vi "UHR-Fleezers Control (host) - 10.4.vi"() -> ()   [LabVIEW 2011] (continued)
        n819 = Select(t=w1240, s="+ phase (GI)", f="Phase adj. (GI)") -> (s? t:f=w1239:i16)
        n820 = Or(x="+ phase (GI)", y="- phase (GI)") -> (x .or. y?=w1235:bool)
        n821 = xnode "Read/Write Control"("FPGA VI Reference In"=w1242, "error in"=w1241, "Phase count adjustment (GI)"=w1239) -> ("FPGA VI Reference Out"=w1237:T19, "error out"=w1238:errorcluster)
        n822 = xnode "Read/Write Control"("FPGA VI Reference In"=w1237, "error in"=w1238, "+ phase (GI)"=w1235) -> ("error out"=w1236:errorcluster)  [unwired: 1 out]
      }
      event "Phase adj. (GI) 2", "+ phase (GI) 2", "- phase (GI) 2": Value Change {
        n823 = event-data() -> ()  [unwired: 7 out]
        n824 = Negate(x="Phase adj. (GI) 2") -> (-x=w1251:i16)
        n825 = Select(t=w1251, s="+ phase (GI) 2", f="Phase adj. (GI) 2") -> (s? t:f=w1250:i16)
        n826 = Or(x="+ phase (GI) 2", y="- phase (GI) 2") -> (x .or. y?=w1246:bool)
        n827 = xnode "Read/Write Control"("FPGA VI Reference In"=w1253, "error in"=w1252, "Phase count adjustment (GI) 2"=w1250) -> ("FPGA VI Reference Out"=w1248:T19, "error out"=w1249:errorcluster)
        n828 = xnode "Read/Write Control"("FPGA VI Reference In"=w1248, "error in"=w1249, "+ phase (GI) 2"=w1246) -> ("error out"=w1247:errorcluster)  [unwired: 1 out]
      }
      event "Phase adj. (Green FB)", "- phase (Green FB)", "+ phase (Green FB)": Value Change {
        n829 = event-data() -> ()  [unwired: 7 out]
        n830 = Negate(x="Phase adj. (Green FB)") -> (-x=w1262:i16)
        n831 = Select(t=w1262, s="+ phase (Green FB)", f="Phase adj. (Green FB)") -> (s? t:f=w1261:i16)
        n832 = Or(x="+ phase (Green FB)", y="- phase (Green FB)") -> (x .or. y?=w1257:bool)
        n833 = xnode "Read/Write Control"("FPGA VI Reference In"=w1264, "error in"=w1263, "Phase count adjustment (Green FB)"=w1261) -> ("FPGA VI Reference Out"=w1259:T19, "error out"=w1260:errorcluster)
        n834 = xnode "Read/Write Control"("FPGA VI Reference In"=w1259, "error in"=w1260, "+ phase (Green FB)"=w1257) -> ("error out"=w1258:errorcluster)  [unwired: 1 out]
      }
      event "Invert APD Gate", "APD Gate ON Count", "APD Gate OFF Count", "APD Gate", "APD Integration Time (s)", "APD 1 AO Mult.", "APD 2 AO Mult.", "On one out of X cycles": Value Change {
        n835 = event-data() -> ()  [unwired: 7 out]
        n836 = Add(x="GI Frequency, ON count", y="GI Frequency, OFF count") -> (x+y=w1268:u32)
        n837 = Add(x="APD Gate ON Count", y="APD Gate OFF Count") -> (x+y=w1281:u32)
        n838 = Multiply(x="On one out of X cycles", y=w1268) -> (x*y=w1265:u32)
        "Green FB Count" <- w1265
        n839 = Subtract(x=w1265, y="GI Frequency, ON count") -> (x-y=w1266:u32)
        n840 = Multiply(x=w1281, y="On one out of X cycles") -> (x*y=w1280:u32)
        n841 = Subtract(x=w1280, y="APD Gate ON Count") -> (x-y=w1279:u32)
        n842 = local read "DMA Update Period (s)"() -> (w1282:dbl)
        n843 = Multiply(x="APD Integration Time (s)", y=40000000.0) -> (x*y=w1287:dbl)
        n844 = Reciprocal(x="APD Integration Time (s)") -> (1/x=→"APD Acq Rate (Hz)":dbl)
        n845 = To Unsigned Long Integer(number=w1287) -> (unsigned 32bit integer=w1271:u32)
        "APD Int. Count" <- w1271
        n846 = xnode "Read/Write Control"("FPGA VI Reference In"=w1291, "error in"=w1290, "Invert APD Gate"="Invert APD Gate", "APD Gate ON Count"="APD Gate ON Count", "APD Gate OFF Count"=w1279, "APD Acq Rate Count"=w1271, "APD Gate Operating Mode"="APD Gate", "APD 1 AO scale factor"="APD 1 AO Mult.", "APD 2 AO scale factor"="APD 2 AO Mult.", "Green interlace ON count"="GI Frequency, ON count", "Green interlace OFF count"=w1266, "Green interlace ON count 2"="GI Frequency, ON count", "Green interlace OFF count 2"=w1266, "Green FB Count"=w1265) -> ("error out"=w1289:errorcluster)  [unwired: 1 out]
        n847 = Divide(x=w1282, y="APD Integration Time (s)") -> (x/y=w1285:dbl)
        n848 = Multiply(x=2.0, y=w1285) -> (x*y=w1284:dbl)
        n849 = local write "APD Samples/FIFO Acq."(w1285) -> ()
        n850 = local write "APD Elements/DMA read"(w1284) -> ()
      }
      event "Number of F/B Scans (AOD)", "Scan Speed (nm/s)", "Scan BD", "Initial delta (MHz)", "Step Size (nm)", "Scan Range (nm)": Value Change {
        w1353 = 123.0  # AOM cal (nm/MHz)
        n851 = event-data() -> ()  [unwired: 7 out]
        n852 = local read "BD 1 Frequency 1 (MHz)"() -> (w1336:dbl)
        n853 = local read "AOM X Cal (nm/MHz)"() -> (w1328:dbl)
        n854 = local read "X RF Frequency Limits (MHz)"() -> (w1340:T16)
        n855 = local read "Y RF Frequency Limits (MHz)"() -> (w1337:T16)
        n856 = local read "BD 2 Frequency 1 (MHz)"() -> (w1342:dbl)
        n857 = Negate(x="Scan Range (nm)") -> (-x=w1306:dbl)
        n858 = Divide(x=w1306, y=w1328) -> (x/y=w1310:dbl)
        n859 = Select(t=w1340, s="Scan BD", f=w1337) -> (s? t:f=w1339:T16)
        n860 = Select(t=w1336, s="Scan BD", f=w1342) -> (s? t:f=w1341:dbl)
        n861 = Unbundle By Name(w1339) -> ("Maximum"=w1348:dbl, "Minimum"=w1347:dbl)
        n862 = Add(x=w1310, y=w1341) -> (x+y=w1345:dbl)
        n863 = Divide(x=w1306, y="Step Size (nm)") -> (x/y=w1325:dbl)
        n864 = Divide(x="Step Size (nm)", y=w1328) -> (x/y=w1334:dbl)
        n865 = Absolute Value(x=w1325) -> (abs(x)=w1309:dbl)
        n866 = Sign(1:w1306) -> (0:w1307:dbl)
        n867 = In Range and Coerce(upper limit=w1348, x=w1345, lower limit=w1347) -> (coerced(x)=w1344:dbl, In Range?=w1346:bool)
        n868 = To Unsigned Quad Integer(1:w1309) -> (0:w1324:u64)
        "Scan steps (AOD)" <- w1324
        n869 = call "IR AOM freq to word.vi"("Frequency In (MHz)"=w1334) -> ("Frequency Word Out (double)"=w1331:dbl)
        n870 = Multiply(x=w1307, y=w1331) -> (x*y=w1308:dbl)
        n871 = Subtract(x=w1345, y=w1344) -> (x-y=w1343:dbl)
        n872 = To Quad Integer(1:w1308) -> (0:w1330:i64)
        "Incr. int (AOD)" <- w1330
        n873 = Subtract(x=w1310, y=w1343) -> (x-y=w1329:dbl)
        "Scan Range (MHz)" <- w1329
        n874 = Select(t=w1310, s=w1346, f=w1329) -> (s? t:f=w1349:dbl)
        n875 = Multiply(x=w1329, y=w1328) -> (x*y=w1327:dbl)
        n876 = Decrement(x=w1324) -> (x-1=w1377:u64)
        n877 = Negate(x=w1327) -> (-x=w1323:dbl)
        n878 = local write "Scan Range (nm)"(w1323) -> ()
        n879 = Divide(x=w1349, y=w1377) -> (x/y=w1333:dbl)
        "Scan Increment (MHz)" <- w1333
        n880 = call "IR AOM freq to word.vi"("Frequency In (MHz)"=w1333) -> ("Frequency Word Out (double)"=w1332:dbl)
        n881 = Divide(x="Step Size (nm)", y="Scan Speed (nm/s)") -> (x/y=w1320:dbl)
        n882 = To Quad Integer(1:w1332) -> ()  [unwired: 1 out]
        n883 = local read "Number Interlace Sets"() -> (w1304:u8)
        n884 = local read "AI Count (ticks)"() -> (w1305:u32)
        n885 = local read "Total Counts (ticks)"() -> (w1303:u32)
        n886 = local read "# Samples/trap"() -> (w1335:u32)
        n887 = Multiply(x=w1305, y=w1304) -> (x*y=w1302:u32)
        n888 = Divide(x=w1303, y=w1302) -> (x/y=w1301:dbl)
        n889 = Select(t=w1336, s="Scan BD", f=w1342) -> (s? t:f=w1374:dbl)
        "Initial freq. (MHz)" <- w1374
        n890 = Add(x=w1349, y=w1374) -> (x+y=→"Final freq. (MHz)":dbl)
        n891 = Divide(x=w1303, y=40000000.0) -> (x/y=w1319:dbl)
        n892 = Divide(x=w1320, y=w1319) -> (x/y=w1318:dbl)
        n893 = To Unsigned Quad Integer(1:w1318) -> (0:w1293:u64)
        n894 = Quotient & Remainder(x=w1293, y=u64 2) -> (x-y*floor(x/y)=w1297:u64)  [unwired: 1 out]
        n895 = Equal?(x=w1297, y=u64 0) -> (x = y?=w1295:bool)
        n896 = Decrement(x=w1293) -> (x-1=w1294:u64)
        n897 = Select(t=w1293, s=w1295, f=w1294) -> (s? t:f=w1292:u64)
        "Cycles/step (AOD)" <- w1292
        n898 = xnode "Read/Write Control"("FPGA VI Reference In"=w1385, "error in"=w1384, "Scan steps"=w1324, "Number of scans"="Number of F/B Scans (AOD)", "Cycles per step"=w1292, "Scan freq.  increment"=w1330, "Scan BD"="Scan BD") -> ("error out"=w1383:errorcluster)  [unwired: 1 out]
        n899 = Multiply(x=w1324, y=w1292) -> (x*y=w1378:u64)
        n900 = Multiply(x=w1378, y=u64 2) -> (x*y=w1300:u64)
        n901 = Multiply(x=w1301, y=w1300) -> (x*y=w1299:dbl)
        "Data points/scan (f/b)" <- w1299
        n902 = Multiply(x=w1299, y="Number of F/B Scans (AOD)") -> (x*y=w1381:dbl)
        "Data points/scans" <- w1381
        n903 = Divide(x=w1381, y=w1335) -> (x/y=→"N sets should be saved":dbl)
        n904 = Multiply(x=w1378, y=w1319) -> (x*y=w1317:dbl)
        "Time/Scan (s) (AOD)" <- w1317
        n905 = Select(t=w1349, s="Scan BD", f=0.0) -> (s? t:f=w1375:dbl)
        n906 = Select(t=0.0, s="Scan BD", f=w1349) -> (s? t:f=w1371:dbl)
        n907 = local read "BD 2 Frequency 2 (MHz)"() -> (w1367:dbl)
        n908 = local read "BD 1 Frequency 2 (MHz)"() -> (w1370:dbl)
        n909 = Add(x=w1371, y=w1342) -> (x+y=w1368:dbl)
        n910 = Add(x=w1336, y=w1375) -> (x+y=w1369:dbl)
        n911 = Multiply(x=w1317, y=2.0) -> (x*y=w1316:dbl)
        n912 = Multiply(x=w1316, y="Number of F/B Scans (AOD)") -> (x*y=w1313:dbl)
        n913 = Divide(x=w1313, y=60.0) -> (x/y=→"Time to Finish All (min)":dbl)
        n914 = Add(x="Trap 2 Bead Size (nm)", y="Trap 1 Bead Size (nm)") -> (x+y=w1357:dbl)
        n915 = Divide(x=w1357, y=2.0) -> (x/y=w1351:dbl)
        n916 = local read "Initial delta (MHz)"() -> (w1354:dbl)
        n917 = Subtract(x=w1368, y=w1367) -> (x-y=w1365:dbl)
        n918 = Subtract(x=w1369, y=w1370) -> (x-y=w1366:dbl)
        n919 = Square(x=w1365) -> (x^2=w1364:dbl)
        n920 = Square(x=w1366) -> (x^2=w1363:dbl)
        n921 = Add(x=w1363, y=w1364) -> (x+y=w1362:dbl)
        n922 = Square Root(x=w1362) -> (sqrt(x)=w1361:dbl)
        "Final delta (MHz)" <- w1361
        n923 = Multiply(x=w1353, y=w1361) -> (x*y=w1360:dbl)
        n924 = Multiply(x=w1354, y=w1353) -> (x*y=w1352:dbl)
        n925 = Subtract(x=w1352, y=w1351) -> (x-y=→"Initial sep (nm)":dbl)
        n926 = Subtract(x=w1360, y=w1351) -> (x-y=→"Final sep (nm)":dbl)
      }
      event "Freq or Amp switch first", "Swap F1 and F2", "Freq switch delay", "Amp switch delay": Value Change {
        n927 = event-data() -> ()  [unwired: 7 out]
        n928 = local read "Freq or Amp switch first"() -> (w1386:bool)
        n929 = local read "Amp switch delay"() -> (w1387:u16)
        n930 = local read "Freq switch delay"() -> (w1389:u16)
        n931 = local read "Swap F1 and F2"() -> (w1388:bool)
        n932 = xnode "Read/Write Control"("FPGA VI Reference In"=w1392, "error in"=w1391, "Freq switch delay"=w1389, "Swap F1 and F2"=w1388, "Amp switch delay"=w1387, "Freq or Amp switch first"=w1386) -> ("error out"=w1390:errorcluster)  [unwired: 1 out]
      }
      event "Scan steps (MCL)", "Number of scans (MCL)", "Scan Range (V)\n(of steps)", "2D or 1D Scan", "N APD Samp/step", "Fast Scan Dir", "Continuous MCL Scanning", "Scan lines (y)": Value Change {
        w1394 = 32767.0 ("y")
        n933 = event-data() -> ()  [unwired: 7 out]
        n934 = Select(t="Scan lines (y)", s="2D or 1D Scan", f="Number of scans (MCL)") -> (s? t:f=w1399:u64)
        n935 = Decrement(x="Scan steps (MCL)") -> (x-1=w1415:u64)
        n936 = Divide(x="Scan Range (V)\n(of steps)", y=w1415) -> (x/y=w1414:dbl)
        "Desired Scan Incr (V)" <- w1414
        n937 = local read "APD Integration Time (s)"() -> (w1407:dbl)
        n938 = Multiply(x=w1414, y=w1394) -> (x*y=w1423:dbl)
        n939 = Divide(x=w1423, y=10.0) -> (x/y=w1413:dbl)
        "Desired incr (int)" <- w1413
        n940 = local read "Update Count (MCL)"() -> (w1419:u32)
        n941 = Round Toward -Infinity(1:w1413) -> (0:w1422:dbl)
        n942 = To Word Integer(number=w1422) -> (16bit integer=w1397:i16)
        "Actual Incr. int (MCL)" <- w1397
        n943 = Multiply(x=w1407, y=40000000.0) -> (x*y=w1420:dbl)
        n944 = Divide(x=w1420, y=w1419) -> (x/y=w1418:dbl)
        n945 = Multiply(x=i16 10, y=w1397) -> (x*y=w1395:i16)
        n946 = Multiply(x="N APD Samp/step", y=w1418) -> (x*y=w1417:dbl)
        "Cycles/step (MCL)" <- w1417
        n947 = Divide(x=w1395, y=w1394) -> (x/y=→"Actual MCL Inc (V)":dbl)
        n948 = Multiply(x="N APD Samp/step", y="Scan steps (MCL)") -> (x*y=w1409:dbl)
        n949 = local read "APD Samples/FIFO Acq."() -> (w1406:dbl)
        n950 = Multiply(x=w1409, y=u64 2) -> (x*y=w1408:dbl)
        "Data points/scan (f+b)" <- w1408
        n951 = Multiply(x=w1408, y=w1399) -> (x*y=w1426:dbl)
        "Data points/scans (MCL)" <- w1426
        n952 = Multiply(x=w1407, y=w1408) -> (x*y=w1400:dbl)
        "Time/f+b scan (s) (MCL)" <- w1400
        n953 = Divide(x=w1426, y=w1406) -> (x/y=→"N sets should be saved (MCL)":dbl)
        n954 = Multiply(x=w1400, y=w1399) -> (x*y=→"Total Time (s)":dbl)
        n955 = Not(x="Fast Scan Dir") -> (.not. x?=w1404:bool)
        n956 = xnode "Read/Write Control"("FPGA VI Reference In"=w1430, "error in"=w1429, "Scan steps (MCL)"="Scan steps (MCL)", "Number of scans (MCL)"=w1399, "Cycles per step (MCL)"=w1417, "Scan freq.  increment (MCL)"=w1397, "1D or 2D Scan?"="2D or 1D Scan", "MCL Scan Axis"=w1404, "Cont. Scan (MCL)"="Continuous MCL Scanning") -> ("error out"=w1428:errorcluster)  [unwired: 1 out]
      }
      event "Read Cal": Value Change {
        w1432 = 1000.0 ("y")
        n957 = event-data() -> ()  [unwired: 7 out]
        n958 = local read "Save file name"() -> (w1457:path)
        n959 = local write "Read Cal"(FALSE ("Read Cal")) -> ()
        n960 = Strip Path(path=w1457) -> (stripped path=w1456:path)  [unwired: 1 out]
        n961 = Path To String(path=w1456) -> (string=w1455:string)
        n962 = Concatenate Strings(w1455, "\\current.cal" ("string")) -> (w1453:string)
        n963 = String To Path(string=w1453) -> (path=w1452:path)
        n964 = Open/Create/Replace File(file path (use dialog)=w1452, operation (0:open)=T25."open", access (0:read/write)=enum16{"read/write", "read-only", "write-only"}."read-only") -> (refnum out=w1460:refnum<file>, error out=w1446:errorcluster)  [unwired: 1 in, 3 out]
        n965 = Deny Access(4:w1446, 7:w1460) -> (0:w1445:errorcluster, 3:w1451:refnum<file>)  [unwired: 1 out]
        n966 = Read from Binary File(5:0.0, 8:w1445, 9:T24."big-endian, network order" ("byte order (0:big-endian, network order)"), 10:-1 ("count (1)"), 11:w1451) -> (0:w1444:errorcluster, 2:w1442:dbl[], 3:w1447:refnum<file>)  [unwired: 2 out]
        n967 = Array To Cluster(array=w1442) -> (cluster=w1441:T27)
        n968 = Unbundle(w1441) -> ("[0]"=w1440:dbl, "[1]"=w1439:dbl, "[2]"=w1438:dbl, "[3]"=w1437:dbl, "[4]"=w1436:dbl, "[5]"=w1435:dbl)
        n969 = Close File(refnum=w1447, error in=w1444) -> (error out=→"Read cal error":errorcluster)  [unwired: 1 out]
        n970 = Multiply(x=w1435, y=w1432) -> (x*y=w1433:dbl)
        n971 = local write "T2 kappa_x (pN/nm)"(w1437) -> ()
        n972 = local write "T1 kappa_x (pN/nm)"(w1438) -> ()
        n973 = local write "T1 alpha_x (nm/V)"(w1440) -> ()
        n974 = local write "T2 alpha_x (nm/V)"(w1439) -> ()
        n975 = Multiply(x=w1436, y=w1432) -> (x*y=w1434:dbl)
        n976 = local write "T1 offset_x (mV)"(w1434) -> ()
        n977 = local write "T2 offset_x (mV)"(w1433) -> ()
      }
      event "Abort MCL Scan": Value Change {
        n978 = event-data() -> ()  [unwired: 7 out]
        n979 = local write "MCL Scanning"(FALSE ("MCL Scanning")) -> ()
        n980 = xnode "Read/Write Control"("FPGA VI Reference In"=w1465, "error in"=w1464, "Abort scan (MCL)"="Abort MCL Scan") -> ("error out"=w1463:errorcluster)  [unwired: 1 out]
      }
      event "Update Count (MCL)": Value Change {
        n981 = event-data() -> ()  [unwired: 7 out]
        n982 = xnode "Read/Write Control"("FPGA VI Reference In"=w1469, "error in"=w1468, "MCL count"="Update Count (MCL)") -> ("error out"=w1467:errorcluster)  [unwired: 1 out]
      }
      event "Phase adjust (MCL)", "+ phase (MCL)", "- phase (MCL)": Value Change {
        n983 = event-data() -> ()  [unwired: 7 out]
        n984 = Negate(x="Phase adjust (MCL)") -> (-x=w1478:i16)
        n985 = Select(t=w1478, s="- phase (MCL)", f="Phase adjust (MCL)") -> (s? t:f=w1476:i16)
        n986 = Or(x="- phase (MCL)", y="+ phase (MCL)") -> (x .or. y?=w1471:bool)
        n987 = xnode "Read/Write Control"("FPGA VI Reference In"=w1480, "error in"=w1479, "Phase count adjustment (MCL)"=w1476) -> ("FPGA VI Reference Out"=w1472:T19, "error out"=w1473:errorcluster)
        n988 = xnode "Read/Write Control"("FPGA VI Reference In"=w1472, "error in"=w1473, "+ phase (MCL)"=w1471) -> ("error out"=w1470:errorcluster)  [unwired: 1 out]
      }
      event "Abort AOD Scan": Value Change {
        n989 = event-data() -> ()  [unwired: 7 out]
        n990 = xnode "Read/Write Control"("FPGA VI Reference In"=w1484, "error in"=w1483, "Abort scan"="Abort AOD Scan") -> ("error out"=w1482:errorcluster)  [unwired: 1 out]
      }
      event "Continuous AOD Scanning": Value Change {
        n991 = event-data() -> ()  [unwired: 7 out]
        n992 = xnode "Read/Write Control"("FPGA VI Reference In"=w1488, "error in"=w1487, "Cont. Scan"="Continuous AOD Scanning") -> ("error out"=w1486:errorcluster)  [unwired: 1 out]
      }
      event "Index": Value Change {
        n993 = event-data() -> ()  [unwired: 7 out]
        n994 = call "Create new save file.vi"("Insert"="", "Ext"=".dat" ("string"), "Index In"="Index") -> ("Path Out"=→"Save file name":path, "Index Out"=w1489:dbl)
        "Save index" <- w1489
        n995 = local write "Index"(w1489) -> ()
      }
      event "AO1", "AO2": Value Change {
        w1504 = 10.0 ("y")
        w1503 = 32767.0 ("y")
        n996 = event-data() -> ()  [unwired: 7 out]
        n997 = local read "AO2"() -> (w1502:dbl)
        n998 = local read "AO1"() -> (w1499:dbl)
        n999 = Multiply(x=w1499, y=w1503) -> (x*y=w1498:dbl)
        n1000 = Multiply(x=w1502, y=w1503) -> (x*y=w1501:dbl)
        n1001 = Divide(x=w1498, y=w1504) -> (x/y=w1497:dbl)
        n1002 = Divide(x=w1501, y=w1504) -> (x/y=w1500:dbl)
        n1003 = To Word Integer(number=w1497) -> (16bit integer=w1505:i16)
        n1004 = To Word Integer(number=w1500) -> (16bit integer=w1506:i16)
        n1005 = xnode "Read/Write Control"("FPGA VI Reference In"=w1496, "error in"=w1495, "AO1"=w1505, "AO2"=w1506) -> ("error out"=w1494:errorcluster)  [unwired: 1 out]
      }
      event "Inject Pump 1": Value Change {
        n1006 = local read "Chemyx Syringe Pump Serial Port"() -> (w1507:refnum<visa-resource-name>)
        n1007 = event-data() -> ()  [unwired: 7 out]
        n1008 = local read "Pump write delay (ms)"() -> (w1508:dbl)
        n1009 = case shown="False" "Inject Pump 1" {
          tunnel: w1508 -> [w1515 w1529]
          tunnel: w1507 -> [w1512 w1528]
          frame False {
            n1010 = flat-sequence {
              tunnel: w1512 -> [w1516]
              tunnel: [w1516] -> w1513
              tunnel: w1515 -> [_]
              tunnel: [w1519] -> w1514
              tunnel: w1513 -> [w1519]
              tunnel: w1514 -> [w1520]
              tunnel: [w1520] -> w1510
              tunnel: [w1522] -> w1511
              tunnel: w1510 -> [w1522]
              tunnel: w1511 -> [w1524]
              frame #0 {
                n1011 = call "Write to pump.vi"("string"="enter pump1", "VISA resource name"=w1516) -> ()  [unwired: 1 out]
              }
              frame #1 {
                n1012 = Wait (ms)(milliseconds to wait="Pump pause delay (ms)") -> ()  [unwired: 1 out]
              }
              frame #2 {
                n1013 = call "Write to pump.vi"("string"="stop", "VISA resource name"=w1520) -> ()  [unwired: 1 out]
              }
              frame #3 {
                n1014 = Wait (ms)(milliseconds to wait=u32 500) -> ()  [unwired: 1 out]
              }
              frame #4 {
                n1015 = call "Write to pump.vi"("string"="stop", "VISA resource name"=w1524) -> ()  [unwired: 1 out]
              }
            }
          }
          frame True {
            n1016 = flat-sequence {
              tunnel: w1528 -> [w1538]
              tunnel: w1529 -> [w1533]
              tunnel: w1529 -> [w1540]
              tunnel: w1528 -> [w1541]
              tunnel: [w1541] -> w1526
              tunnel: [w1543] -> w1527
              tunnel: w1526 -> [w1543]
              tunnel: w1527 -> [w1545]
              frame #0 {
                n1017 = local read "All Pump Parameters"() -> (w1532:T5)
                n1018 = Unbundle By Name(w1532) -> ("Pump 1"=w1539:T28)
                n1019 = call "Set pump parameters.vi"("Pump write delay (ms)"=w1533, "Volume (uL)"="Ch 1 Inject Volume (uL)", "Rate (uL/h)"="Ch 1 Inject Rate (ul/h)", "Units"=4.0, "Pump #"=1.0, "Pump Parameters In"=w1539, "VISA resource name"=w1538) -> ("Pump Parameters Out"=w1531:T28)  [unwired: 3 in]
                n1020 = Bundle By Name(cluster=w1532, "Pump 1"=w1531) -> (w1530:T5)
                n1021 = local write "All Pump Parameters"(w1530) -> ()
              }
              frame #1 {
                n1022 = Wait (ms)(milliseconds to wait=w1540) -> ()  [unwired: 1 out]
              }
              frame #2 {
                n1023 = call "Write to pump.vi"("string"="start", "VISA resource name"=w1541) -> ()  [unwired: 1 out]
              }
              frame #3 {
                n1024 = Wait (ms)(milliseconds to wait=u32 500) -> ()  [unwired: 1 out]
              }
              frame #4 {
                n1025 = call "Write to pump.vi"("string"="start", "VISA resource name"=w1545) -> ()  [unwired: 1 out]
              }
            }
          }
        }
      }
      event "Inject Pump 3": Value Change {
        n1026 = event-data() -> ()  [unwired: 7 out]
        n1027 = local read "Pump write delay (ms)"() -> (w1548:dbl)
        n1028 = case shown="False" "Inject Pump 3" {
          tunnel: w1548 -> [w1555 w1569]
          tunnel: "Chemyx Syringe Pump Serial Port" -> [w1552 w1568]
          frame False {
            n1029 = flat-sequence {
              tunnel: w1552 -> [w1556]
              tunnel: [w1556] -> w1553
              tunnel: w1555 -> [_]
              tunnel: [w1559] -> w1554
              tunnel: w1553 -> [w1559]
              tunnel: w1554 -> [w1560]
              tunnel: [w1560] -> w1550
              tunnel: [w1562] -> w1551
              tunnel: w1550 -> [w1562]
              tunnel: w1551 -> [w1564]
              frame #0 {
                n1030 = call "Write to pump.vi"("string"="enter pump3", "VISA resource name"=w1556) -> ()  [unwired: 1 out]
              }
              frame #1 {
                n1031 = local read "Pump pause delay (ms)"() -> (w1558:u32)
                n1032 = Wait (ms)(milliseconds to wait=w1558) -> ()  [unwired: 1 out]
              }
              frame #2 {
                n1033 = call "Write to pump.vi"("string"="stop", "VISA resource name"=w1560) -> ()  [unwired: 1 out]
              }
              frame #3 {
                n1034 = Wait (ms)(milliseconds to wait=u32 0) -> ()  [unwired: 1 out]
              }
              frame #4 {
                n1035 = call "Write to pump.vi"("string"="stop", "VISA resource name"=w1564) -> ()  [unwired: 1 out]
              }
            }
          }
          frame True {
            n1036 = flat-sequence {
              tunnel: w1568 -> [w1578]
              tunnel: w1569 -> [w1573]
              tunnel: w1569 -> [w1580]
              tunnel: w1568 -> [w1581]
              tunnel: [w1581] -> w1566
              tunnel: [w1584] -> w1567
              tunnel: w1566 -> [w1584]
              tunnel: w1567 -> [w1585]
              frame #0 {
                n1037 = local read "All Pump Parameters"() -> (w1572:T5)
                n1038 = Unbundle By Name(w1572) -> ("Pump 3"=w1579:T28)
                n1039 = call "Set pump parameters.vi"("Pump write delay (ms)"=w1573, "Volume (uL)"="Ch 3 Inject Volume (uL)", "Rate (uL/h)"="Ch 3 Inject Rate (ul/h)", "Units"=4.0, "Pump #"=3.0, "Pump Parameters In"=w1579, "VISA resource name"=w1578) -> ("Pump Parameters Out"=w1571:T28)  [unwired: 3 in]
                n1040 = Bundle By Name(cluster=w1572, "Pump 3"=w1571) -> (w1570:T5)
                n1041 = local write "All Pump Parameters"(w1570) -> ()
              }
              frame #1 {
                n1042 = Wait (ms)(milliseconds to wait=w1580) -> ()  [unwired: 1 out]
              }
              frame #2 {
                n1043 = call "Write to pump.vi"("string"="start", "VISA resource name"=w1581) -> ()  [unwired: 1 out]
              }
              frame #3 {
                n1044 = Wait (ms)(milliseconds to wait=u32 500) -> ()  [unwired: 1 out]
              }
              frame #4 {
                n1045 = call "Write to pump.vi"("string"="start", "VISA resource name"=w1585) -> ()  [unwired: 1 out]
              }
            }
          }
        }
      }
      event "Inject Pump 2": Value Change {
        n1046 = event-data() -> ()  [unwired: 7 out]
        n1047 = local read "Pump write delay (ms)"() -> (w1589:dbl)
        n1048 = flat-sequence {
          tunnel: w1587 -> [w1602]
          tunnel: w1589 -> [w1598]
          tunnel: "Inject Pump 2" -> [_]
          tunnel: w1589 -> [w1604]
          tunnel: w1587 -> [w1605]
          frame #0 {
            n1049 = local read "All Pump Parameters"() -> (w1597:T5)
            n1050 = Multiply(x=60.0, y="Flush Center Ch Rate (ul/m)") -> (x*y=w1594:dbl)
            n1051 = Unbundle By Name(w1597) -> ("Pump 2"=w1603:T28)
            n1052 = call "Set pump parameters.vi"("Pump write delay (ms)"=w1598, "Volume (uL)"="Flush Center Ch Volume (uL)", "Rate (uL/h)"=w1594, "Units"=3.0, "Pump #"=2.0, "Pump Parameters In"=w1603, "VISA resource name"=w1602) -> ("Pump Parameters Out"=w1596:T28)  [unwired: 3 in]
            n1053 = Bundle By Name(cluster=w1597, "Pump 2"=w1596) -> (w1595:T5)
            n1054 = local write "All Pump Parameters"(w1595) -> ()
            n1055 = Add(x="Flush Center Ch Volume (uL)", y="Total Volume\nFlushed (uL)") -> (x+y=w1591:dbl)
            n1056 = local write "Total Volume\nFlushed (uL)"(w1591) -> ()
          }
          frame #1 {
            n1057 = Wait (ms)(milliseconds to wait=w1604) -> ()  [unwired: 1 out]
          }
          frame #2 {
            n1058 = call "Write to pump.vi"("string"="start", "VISA resource name"=w1605) -> ()  [unwired: 1 out]
          }
        }
        n1059 = local read "Chemyx Syringe Pump Serial Port"() -> (w1587:refnum<visa-resource-name>)
      }
      event "Sample Channel\nFlow": Value Change {
        n1060 = event-data() -> ()  [unwired: 7 out]
        n1061 = case shown="True" "Sample Channel\nFlow" {
          tunnel: w1609 -> [w1615 w1617]
          tunnel: [w1615 w1616] -> w1608
          frame False {
          }
          frame True {
            n1062 = Number To Decimal String(number="Flow rate (uL/h)") -> (decimal integer string=w1622:string)  [unwired: 1 in]
            n1063 = Concatenate Strings("irate  " ("string"), w1622, " u/h" ("string"), "\r") -> (w1620:string)
            n1064 = VISA Write(VISA resource name=w1617, write buffer=w1620) -> (VISA resource name out=w1616:refnum<visa-resource-name>)  [unwired: 1 in, 2 out]
          }
        }
        n1065 = Select(t="run" ("string"), s="Sample Channel\nFlow", f="stop" ("string")) -> (s? t:f=w1610:string)
        n1066 = Concatenate Strings(w1610, "\r") -> (w1613:string)
        n1067 = VISA Write(VISA resource name=w1608, write buffer=w1613) -> ()  [unwired: 1 in, 3 out]
      }
      event "Flow rate (uL/h)": Value Change {
        n1068 = event-data() -> ()  [unwired: 7 out]
        n1069 = local read "Flow rate (uL/h)"() -> (w1626:dbl)
        n1070 = Number To Decimal String(number=w1626) -> (decimal integer string=w1629:string)  [unwired: 1 in]
        n1071 = Concatenate Strings("irate  " ("string"), w1629, " u/h" ("string"), "\r") -> (w1628:string)
        n1072 = VISA Write(VISA resource name=w1624, write buffer=w1628) -> ()  [unwired: 1 in, 3 out]
      }
      event "Flush Sample": Value Change {
        n1073 = event-data() -> ()  [unwired: 7 out]
        n1074 = Number To Decimal String(number="Flush rate (uL/m)") -> (decimal integer string=w1648:string)  [unwired: 1 in]
        n1075 = Concatenate Strings("irate  " ("string"), w1648, " u/m" ("string"), "\r") -> (w1650:string)
        n1076 = VISA Write(VISA resource name=w1652, write buffer=w1650) -> (VISA resource name out=w1646:refnum<visa-resource-name>)  [unwired: 1 in, 2 out]
        n1077 = Number To Decimal String(number="Volume (uL)") -> (decimal integer string=w1635:string)  [unwired: 1 in]
        n1078 = Concatenate Strings("tvolume  " ("string"), w1635, " u" ("string"), "\r") -> (w1633:string)
        n1079 = VISA Write(VISA resource name=w1646, write buffer=w1633) -> (VISA resource name out=w1632:refnum<visa-resource-name>)  [unwired: 1 in, 2 out]
        n1080 = Concatenate Strings("cvolume" ("string"), "\r") -> (w1631:string)
        n1081 = VISA Write(VISA resource name=w1632, write buffer=w1631) -> (VISA resource name out=w1644:refnum<visa-resource-name>)  [unwired: 1 in, 2 out]
        n1082 = Concatenate Strings("run" ("string"), "\r") -> (w1642:string)
        n1083 = VISA Write(VISA resource name=w1644, write buffer=w1642) -> ()  [unwired: 1 in, 3 out]
      }
      event "Clear Volume": Value Change {
        n1084 = event-data() -> ()  [unwired: 7 out]
        n1085 = Concatenate Strings("cvolume" ("string"), "\r") -> (w1655:string)
        n1086 = VISA Write(VISA resource name=w1654, write buffer=w1655) -> ()  [unwired: 1 in, 3 out]
      }
      event "Flip Green Filter": Value Change {
        n1087 = event-data() -> ()  [unwired: 7 out]
        n1088 = Not(x="Flip Green Filter") -> (.not. x?=w1659:bool)
        n1089 = local write "Flip Green Filter"(w1659) -> ()
        n1090 = flat-sequence {
          tunnel: w1667 -> [w1672]
          tunnel: w1666 -> [w1671]
          tunnel: [w1669] -> w1664
          tunnel: [w1668] -> w1663
          tunnel: [w1674] -> w1662
          tunnel: w1664 -> [w1674]
          tunnel: [w1673] -> w1661
          tunnel: w1663 -> [w1673]
          tunnel: w1662 -> [w1678]
          tunnel: w1661 -> [w1677]
          tunnel: [w1676] -> w1665
          frame #0 {
            n1091 = xnode "Read/Write Control"("FPGA VI Reference In"=w1672, "error in"=w1671, "Green Filter Flipper"=TRUE) -> ("FPGA VI Reference Out"=w1669:T19, "error out"=w1668:errorcluster)
          }
          frame #1 {
            n1092 = Wait (ms)(milliseconds to wait=u32 100) -> ()  [unwired: 1 out]
          }
          frame #2 {
            n1093 = xnode "Read/Write Control"("FPGA VI Reference In"=w1678, "error in"=w1677, "Green Filter Flipper"=FALSE) -> ("error out"=w1676:errorcluster)  [unwired: 1 out]
          }
        }
      }
      event "Pump 1 contents", "Pump 3 contents": Value Change {
        n1094 = event-data() -> ()  [unwired: 7 out]
        n1095 = local read "Pump 1 contents"() -> (→"Pump 1 cont disp":string)
        n1096 = local read "Pump 3 contents"() -> (→"Pump 3 cont disp":string)
      }
      event "Reset Trap Pos. FB": Value Change {
        n1097 = event-data() -> ()  [unwired: 7 out]
        n1098 = xnode "Read/Write Control"("FPGA VI Reference In"=w1684, "error in"=w1683, "Trap Pos. FB Reset"="Reset Trap Pos. FB") -> ()  [unwired: 2 out]
      }
      event "Rem fb disp offset": Value Change {
        n1099 = event-data() -> ()  [unwired: 7 out]
        n1100 = local write "Rem fb disp offset"(FALSE ("Rem fb disp offset")) -> ()
        n1101 = local read "Mean T1 Position (nm)"() -> (w1686:dbl)
        n1102 = local read "FB Trap Pos Offset"() -> (w1687:dbl)
        n1103 = Subtract(x=w1687, y=w1686) -> (x-y=w1685:dbl)
        n1104 = local write "FB Trap Pos Offset"(w1685) -> ()
      }
      event "Threshold (nm)": Value Change {
        n1105 = event-data() -> ()  [unwired: 7 out]
        n1106 = flat-sequence {
          tunnel: w1691 -> [w1699]
          tunnel: w1690 -> [w1698]
          tunnel: [w1692] -> w1689
          tunnel: w1689 -> [w1705]
          frame #0 {
            n1107 = xnode "Read/Write Control"("FPGA VI Reference In"=w1699, "error in"=w1698) -> ("FPGA VI Reference Out"=w1695:T19, "error out"=w1694:errorcluster, "FPGA TTrig Thresh"=w1696:i64)
            n1108 = local read "Threshold stored (nm)"() -> (w1704:dbl)
            n1109 = local read "Threshold (nm)"() -> (w1692:dbl)
            n1110 = local read "AOM X Cal (nm/MHz)"() -> (w1702:dbl)
            n1111 = Subtract(x=w1692, y=w1704) -> (x-y=w1703:dbl)
            n1112 = Divide(x=w1703, y=w1702) -> (x/y=w1700:dbl)
            n1113 = call "IR AOM freq to word.vi"("Frequency In (MHz)"=w1700) -> ("Frequency Word Out (double)"=w1701:dbl)
            n1114 = To Quad Integer(1:w1701) -> (0:w1697:i64)
            n1115 = Add(x=w1696, y=w1697) -> (x+y=w1693:i64)
            n1116 = xnode "Read/Write Control"("FPGA VI Reference In"=w1695, "error in"=w1694, "FPGA TTrig Thresh"=w1693) -> ()  [unwired: 2 out]
          }
          frame #1 {
            "Threshold stored (nm)" <- w1705
          }
        }
      }
      event "FB Trig Integrate": Value Change {
        n1117 = event-data() -> ()  [unwired: 7 out]
        n1118 = local read "FB Trig Integrate"() -> (w1707:u32)
        n1119 = xnode "Read/Write Control"("FPGA VI Reference In"=w1709, "error in"=w1708, "FB Trig Integrate"=w1707) -> ("error out"=w1706:errorcluster)  [unwired: 1 out]
      }
      event "11": Value Change {
        n1120 = event-data() -> ()  [unwired: 7 out]
        n1121 = local read "11"() -> (w1710:bool)
        n1122 = case shown="True" w1710 {
          frame False {
          }
          frame True {
            n1123 = local read "Messages"() -> (w1712:string)
            n1124 = call "Update messages.vi"("Message to add"="You kicked it up to 11!", "Old message string"=w1712) -> ("New message string"=w1713:string)
            n1125 = call <vilib>:"Beep.vi"() -> ()  [unwired: 12 in]
            n1126 = local write "Messages"(w1713) -> ()
          }
        }
      }
      event "Trap Pos. FB ON": Value Change {
        n1127 = event-data() -> ()  [unwired: 7 out]
        n1128 = xnode "Read/Write Control"("FPGA VI Reference In"=w1716, "error in"=w1715, "Force feedback"="Trap Pos. FB ON") -> ()  [unwired: 2 out]
      }
      event "Remove Action Offset": Value Change {
        n1129 = event-data() -> ()  [unwired: 7 out]
        n1130 = local write "Remove Action Offset"(FALSE ("Remove Action Offset")) -> ()
        n1131 = local read "Trap Pos. FB Mult Factor"() -> (w1721:i64)
        n1132 = local read "Trap Pos FB Action"() -> (w1719:i64)
        n1133 = local read "Trap Pos. FB Offset Factor"() -> (w1717:i64)
        n1134 = Multiply(x=w1721, y=w1719) -> (x*y=w1720:i64)
        n1135 = Add(x=w1720, y=w1717) -> (x+y=w1718:i64)
        n1136 = local write "Trap Pos. FB Offset Factor"(w1718) -> ()
        n1137 = xnode "Read/Write Control"("FPGA VI Reference In"=w1724, "error in"=w1723, "Trap Pos. FB Offset Factor"=w1718) -> ()  [unwired: 2 out]
      }
      event "Remove Unwinding Offset": Value Change {
        n1138 = event-data() -> ()  [unwired: 7 out]
        n1139 = local write "Remove Unwinding Offset"(FALSE ("Remove Action Offset")) -> ()
        n1140 = local read "Trap Pos. FB Mult Factor"() -> (w1736:i64)
        n1141 = local read "Trap Pos FB Action"() -> (w1734:i64)
        n1142 = local read "Trap Pos. FB Offset Factor"() -> (w1733:i64)
        n1143 = Multiply(x=w1736, y=w1734) -> (x*y=w1735:i64)
        n1144 = local read "Trap Pos. FB Mult Factor"() -> (w1732:i64)
        n1145 = Add(x=w1735, y=w1733) -> (x+y=w1726:i64)
        n1146 = Multiply(x=32768, y="factor") -> (x*y=w1729:dbl)
        n1147 = Multiply(x=w1729, y=w1732) -> (x*y=w1731:dbl)
        n1148 = Subtract(x=w1726, y=w1731) -> (x-y=w1730:dbl)
        n1149 = To Quad Integer(1:w1730) -> (0:w1725:i64)
        n1150 = xnode "Read/Write Control"("FPGA VI Reference In"=w1739, "error in"=w1738, "Trap Pos. FB Offset Factor"=w1725) -> ()  [unwired: 2 out]
        n1151 = local write "Trap Pos. FB Offset Factor"(w1725) -> ()
      }
      event "Trap Pos. FB Range", "Trap Pos. FB Gains", "Trap Pos. FB Mult Factor", "Trap Pos. FB Offset Factor", "Trap Pos FB Negate Action", "Trap Pos FB Monitor\nT1 or T2": Value Change {
        n1152 = event-data() -> ()  [unwired: 7 out]
        n1153 = xnode "Read/Write Control"("FPGA VI Reference In"=w1748, "error in"=w1747, "Trap Pos. FB Range"="Trap Pos. FB Range", "Trap Pos. FB Gains"="Trap Pos. FB Gains", "Trap Pos. FB Mult Factor"="Trap Pos. FB Mult Factor", "Trap Pos. FB Offset Factor"="Trap Pos. FB Offset Factor", "Trap Pos FB Negate Action"="Trap Pos FB Negate Action", "Trap Pos FB Monitor T1 or T2"="Trap Pos FB Monitor\nT1 or T2", "AI1 X Scale"="Trap Pos. AI1 X Pre-scale") -> ()  [unwired: 2 out]
      }
      event "Trap Pos FB SP": Value Change {
        n1154 = event-data() -> ()  [unwired: 7 out]
        n1155 = xnode "Read/Write Control"("FPGA VI Reference In"=w1751, "error in"=w1750, "Trap Pos. FB SP"="Trap Pos FB SP") -> ()  [unwired: 2 out]
      }
      event "Set Reading to\nSetpoint": Value Change {
        n1156 = event-data() -> ()  [unwired: 7 out]
        n1157 = local read "Trap Pos FB Monitor\nT1 or T2"() -> (w1760:bool)
        n1158 = local read "Trap X AI1 (DMA)"() -> (w1763:T13)
        n1159 = local write "Set Reading to\nSetpoint"(FALSE ("Set SP to Reading")) -> ()
        n1160 = local read "Trap X (AI1)"() -> (w1766:T10)
        n1161 = Unbundle By Name(w1766) -> ("Trap 1"=w1765:fxp<+/-,16,1>, "Trap 2"=w1764:fxp<+/-,16,1>)
        n1162 = Unbundle By Name(w1763) -> ("Set 1"=w1762:fxp<+/-,16,1>, "Set 2"=w1761:fxp<+/-,16,1>)
        n1163 = Select(t=w1765, s=w1760, f=w1764) -> (s? t:f=w1759:fxp<+/-,16,1>)
        n1164 = Select(t=w1762, s=w1760, f=w1761) -> (s? t:f=w1758:fxp<+/-,16,1>)
        n1165 = Not(x="Set SP Using...") -> (.not. x?=w1753:bool)
        n1166 = Select(t=w1759, s=w1753, f=w1758) -> (s? t:f=w1754:fxp<+/-,16,1>)
        n1167 = xnode "Read/Write Control"("FPGA VI Reference In"=w1756, "error in"=w1755, "Trap Pos. FB SP"=w1754) -> ()  [unwired: 2 out]
        n1168 = local write "Trap Pos FB SP"(w1754) -> ()
      }
      event "Trap Pos. FB Out Scale 2^n": Value Change {
        n1169 = event-data() -> ()  [unwired: 7 out]
        n1170 = Scale By Power Of 2(n="Trap Pos. FB Out Scale 2^n", x=ext 1.0) -> (x*2^n=w1767:ext)
        n1171 = property on="Trap Pos. FB Mult Factor" class="DigNum (strict)"("Val(Sgnl)"=w1767) -> ()  [unwired: 2 in, 2 out]
      }
      event "Trap Pos FB Int Count": Value Change {
        n1172 = event-data() -> ()  [unwired: 7 out]
        n1173 = xnode "Read/Write Control"("FPGA VI Reference In"=w1772, "error in"=w1771, "Trap Pos FB Int Count"="Trap Pos FB Int Count") -> ()  [unwired: 2 out]
      }
    }
    "error out 2" <- w898
    n1174 = node-c288() -> ()  [unwired: 2 out]
  }
  n1175 = disable-structure shown="Disabled" {
    disable-tunnel: [w1774 _] -> w218
    disable-tunnel: w38 -> [w1773 _]
    frame Disabled {
      n1176 = node-c288() -> (w1776:T21)  [unwired: 4 out]
      n1177 = timed-loop "Rough control of MCL mirror stage (debugging)" {
        tunnel: w1773 -> [w1779]
        tunnel: [w1778] -> w1774
        timing: w1776 -> [_]
        timing-out: [_] -> w1775
        stop <- w1778 stop-if-true
        n1178 = node-c288() -> ()  [unwired: 2 out]
        n1179 = case shown="1" "MCL Mode" {
          tunnel: w1779 -> [_ w1782 w1829]
          frame 0, Default {
          }
          frame 1 {
            n1180 = node-c288() -> (w1784:T21)  [unwired: 4 out]
            n1181 = timed-loop "Oscillate MCL mirror" {
              timing: w1784 -> [_]
              timing-out: [_] -> w1783
              tunnel: w1782 -> [w1823]
              i -> [w1822]
              stop <- w1785 stop-if-true
              n1182 = node-c288() -> (w1821:i64)  [unwired: 1 out]
              n1183 = Multiply(x="AO1", y=32767.0) -> (x*y=w1817:dbl)
              n1184 = Multiply(x="AO2", y=32767.0) -> (x*y=w1812:dbl)
              n1185 = Divide(x=w1817, y=10.0) -> (x/y=w1818:dbl)
              n1186 = Divide(x=w1812, y=10.0) -> (x/y=w1813:dbl)
              n1187 = To Word Integer(number=w1818) -> (16bit integer=w1810:i16)
              n1188 = To Word Integer(number=w1813) -> (16bit integer=w1809:i16)
              n1189 = Divide(x=w1821, y=i64 1000) -> (x/y=w1792:dbl)
              n1190 = Multiply(x=w1792, y=w1822) -> (x*y=w1803:dbl)
              n1191 = Multiply(x="Osc. freq. (Hz) 2", y=6.283185307179586) -> (x*y=w1804:dbl)
              n1192 = Multiply(x=w1804, y=w1803) -> (x*y=w1802:dbl)
              n1193 = Sine(x=w1802) -> (sin(x)=w1801:dbl)
              n1194 = Multiply(x=w1801, y="Osc. amp. (V)") -> (x*y=w1799:dbl)
              n1195 = Add(x=w1799, y="Osc. center (V)") -> (x+y=w1797:dbl)
              n1196 = Divide(x=w1797, y=10.0) -> (x/y=w1795:dbl)
              n1197 = Multiply(x=w1795, y=32767.0) -> (x*y=w1790:dbl)
              n1198 = Select(t=w1790, s="Scan axis", f=w1810) -> (s? t:f=w1808:dbl)
              n1199 = Select(t=w1809, s="Scan axis", f=w1790) -> (s? t:f=w1807:dbl)
              n1200 = local read "MCL Mode"() -> (w1789:u16)
              n1201 = Not Equal?(x=w1789, y=u16 1) -> (x != y?=w1786:bool)
              n1202 = local read "Stop All"() -> (w1787:bool)
              n1203 = xnode "Read/Write Control"("FPGA VI Reference In"=w1823, "AO1"=w1808, "AO2"=w1807) -> ()  [unwired: 1 in, 2 out]
              n1204 = Compound Arithmetic op=OR(w1787, w1786) -> (w1785:bool)
              n1205 = node-c288() -> ()  [unwired: 2 out]
            }
            n1206 = node-c288(w1783) -> ()  [unwired: 1 out]
          }
          frame 2 {
            n1207 = case shown="True" "Start Scan" {
              tunnel: w1829 -> [_ w1841]
              frame False {
              }
              frame True {
                n1208 = Subtract(x="End (V)", y="Begin (V)") -> (x-y=w1837:dbl)
                n1209 = Decrement(x="N Points") -> (x-1=w1836:dbl)
                n1210 = Divide(x=w1837, y=w1836) -> (x/y=w1834:dbl)
                n1211 = for {
                  N: "N Points" -> [_]
                  tunnel: "Begin (V)" -> [w1854]
                  tunnel: w1841 -> [w1846]
                  tunnel: [w1845] -> w1840 mode=indexing
                  tunnel: w1834 -> [w1844]
                  tunnel: [w1842] -> w1833 mode=indexing
                  i -> [w1853]
                  n1212 = Multiply(x=w1844, y=w1853) -> (x*y=w1852:dbl)
                  n1213 = Add(x=w1854, y=w1852) -> (x+y=w1849:dbl)
                  n1214 = local read "Scan axis"() -> (w1843:bool)
                  n1215 = local read "AO1"() -> (w1851:dbl)
                  n1216 = local read "AO2"() -> (w1850:dbl)
                  n1217 = Select(t=w1849, s=w1843, f=w1851) -> (s? t:f=w1848:dbl)
                  n1218 = Select(t=w1850, s=w1843, f=w1849) -> (s? t:f=w1847:dbl)
                  n1219 = flat-sequence {
                    tunnel: w1848 -> [w1858]
                    tunnel: w1847 -> [w1857]
                    tunnel: w1846 -> [w1855]
                    tunnel: [w1868] -> w1845
                    tunnel: [w1867] -> w1842
                    frame #0 {
                      w1861 = 10.0 ("y")
                      w1856 = 32767.0 ("y")
                      n1220 = Multiply(x=w1858, y=w1856) -> (x*y=w1864:dbl)
                      n1221 = Multiply(x=w1857, y=w1856) -> (x*y=w1862:dbl)
                      n1222 = Divide(x=w1864, y=w1861) -> (x/y=w1865:dbl)
                      n1223 = Divide(x=w1862, y=w1861) -> (x/y=w1863:dbl)
                      n1224 = To Word Integer(number=w1865) -> (16bit integer=w1859:i16)
                      n1225 = To Word Integer(number=w1863) -> (16bit integer=w1860:i16)
                      n1226 = xnode "Read/Write Control"("FPGA VI Reference In"=w1855, "AO1"=w1859, "AO2"=w1860) -> ()  [unwired: 1 in, 2 out]
                    }
                    frame #1 {
                      n1227 = Wait (ms)(milliseconds to wait="DAQ Delay (ms)") -> ()  [unwired: 1 out]
                    }
                    frame #2 {
                      n1228 = local read "Slow mean"() -> (w1868:dbl)
                      n1229 = local read "Sigma"() -> (w1867:dbl)
                    }
                  }
                }
                n1230 = Bundle("Begin (V)"="Begin (V)", w1834, w1840) -> (→"MCL Scan":cluster{"Begin (V)":dbl, dbl, dbl[]})  [unwired: 1 out]
                n1231 = Bundle("Begin (V)"="Begin (V)", w1834, w1833) -> (→"MCL Scan 2":cluster{"Begin (V)":dbl, dbl, dbl[]})  [unwired: 1 out]
              }
            }
          }
        }
        n1232 = local read "Stop All"() -> (w1778:bool)
        n1233 = node-c288() -> ()  [unwired: 2 out]
      }
      n1234 = node-c288(w1775) -> ()  [unwired: 1 out]
    }
    frame Enabled {
    }
  }
  n1235 = node-c288() -> (w82:T21)  [unwired: 4 out]
  n1236 = node-c288(3 ("Processor")) -> (w78:T21)  [unwired: 3 out]
  n1237 = timed-loop "Mouse control: trap position (AOM deflection), set confocal spot from image" {
    tunnel: [w1872] -> w170
    tunnel: w38 -> [w1871]
    timing: w82 -> [_]
    timing-out: [_] -> w81
    stop <- w1872 stop-if-true
    n1238 = node-c288() -> ()  [unwired: 2 out]
    n1239 = event shown="[0] \"Pane\": Mouse Down" {
      selector: _ -> [_ _]
      dyn-events: _ -> [_ _]
      timeout: _ -> [_ _]
      tunnel: w1871 -> [w1875 _]
      event Mouse Down {
        n1240 = event-data() -> ("Time"=w1877:u32, "Coords"=w1876:T7, "Button"=w1878:u16)  [unwired: 6 out]
        n1241 = case shown="1" w1878 {
          tunnel: w1877 -> [_ _ w1981]
          tunnel: w1876 -> [_ w1915 w1979]
          tunnel: w1875 -> [_ _ w1977]
          frame 0, Default {
          }
          frame 1 {
            n1242 = property on="APD 2" class="ImageControl"() -> ("Displayed Image Position"=w1885:cluster{"Left":i32, "Top":i32})  [unwired: 2 in, 2 out]
            n1243 = property on="APD 1" class="ImageControl"() -> ("Displayed Image Position"=w1914:cluster{"Left":i32, "Top":i32})  [unwired: 2 in, 2 out]
            n1244 = property on="Detection Laser X" class="ImageControl"() -> ("Displayed Image Position"=w1911:cluster{"Left":i32, "Top":i32})  [unwired: 2 in, 2 out]
            n1245 = property on="Detection Laser Y" class="ImageControl"() -> ("Displayed Image Position"=w1910:cluster{"Left":i32, "Top":i32})  [unwired: 2 in, 2 out]
            n1246 = property on="APD 2" class="ImageControl"() -> ("Displayed Image Size"=w1884:cluster{"Width":u32, "Height":u32})  [unwired: 2 in, 2 out]
            n1247 = property on="APD 1" class="ImageControl"() -> ("Displayed Image Size"=w1912:cluster{"Width":u32, "Height":u32})  [unwired: 2 in, 2 out]
            n1248 = property on="Detection Laser X" class="ImageControl"() -> ("Displayed Image Size"=w1913:cluster{"Width":u32, "Height":u32})  [unwired: 2 in, 2 out]
            n1249 = property on="Detection Laser Y" class="ImageControl"() -> ("Displayed Image Size"=w1909:cluster{"Width":u32, "Height":u32})  [unwired: 2 in, 2 out]
            n1250 = Unbundle By Name(w1884) -> ("Width"=w1881:u32, "Height"=w1880:u32)
            n1251 = Unbundle By Name(w1885) -> ("Left"=w1883:i32, "Top"=w1882:i32)
            n1252 = Unbundle By Name(w1912) -> ("Width"=w1906:u32, "Height"=w1905:u32)
            n1253 = Unbundle By Name(w1913) -> ("Width"=w1902:u32, "Height"=w1901:u32)
            n1254 = Unbundle By Name(w1909) -> ("Width"=w1898:u32, "Height"=w1897:u32)
            n1255 = Unbundle By Name(w1914) -> ("Left"=w1908:i32, "Top"=w1907:i32)
            n1256 = Unbundle By Name(w1911) -> ("Left"=w1904:i32, "Top"=w1903:i32)
            n1257 = Unbundle By Name(w1910) -> ("Left"=w1900:i32, "Top"=w1899:i32)
            n1258 = Bundle("Left"=w1883, "Top"=w1882, "Width"=w1881, "Height"=w1880) -> (w1879:T29)  [unwired: 1 in]
            n1259 = Bundle("Left"=w1908, "Top"=w1907, "Width"=w1906, "Height"=w1905) -> (w1896:T29)  [unwired: 1 in]
            n1260 = Bundle("Left"=w1904, "Top"=w1903, "Width"=w1902, "Height"=w1901) -> (w1895:T29)  [unwired: 1 in]
            n1261 = Bundle("Left"=w1900, "Top"=w1899, "Width"=w1898, "Height"=w1897) -> (w1894:T29)  [unwired: 1 in]
            n1262 = Build Cluster Array(w1879, w1896, w1895, w1894) -> (w1893:T30)
            n1263 = for {
              tunnel: w1915 -> [w1926]
              tunnel: w1893 -> [w1927] mode=indexing
              shift-right: [w1924] -> w1891
              shift-left: TRUE -> [w1925]
              shift-right: [w1923] -> w1889
              shift-left: _ -> [w1919]
              shift-right: [w1922] -> w1888
              shift-left: _ -> [w1918]
              shift-right: [w1921] -> w1887
              shift-left: _ -> [w1917]
              shift-right: [w1920] -> w1886
              shift-left: _ -> [w1916]
              n1264 = case shown="True" w1925 {
                selector: w1925 -> [w1932 _]
                tunnel: w1927 -> [_ w1941]
                tunnel: w1926 -> [_ w1939]
                tunnel: [w1932 w1937] -> w1924
                tunnel: [w1931 w1936] -> w1923
                tunnel: [w1930 w1935] -> w1922
                tunnel: [w1929 w1934] -> w1921
                tunnel: [w1928 w1933] -> w1920
                tunnel: w1919 -> [w1931 _]
                tunnel: w1918 -> [w1930 _]
                tunnel: w1917 -> [w1929 _]
                tunnel: w1916 -> [w1928 _]
                frame False {
                }
                frame True {
                  n1265 = Unbundle(w1941) -> (w1940:T29)
                  n1266 = call "isclickinwindow.vi"("Image Param"=w1940, "Point32"=w1939) -> ("4 Y"=w1933:i32, "3 Height"=w1934:i32, "2 X"=w1935:i32, "1 Width"=w1936:i32, "In image?"=w1938:bool)  [unwired: 1 in]
                  n1267 = Not(x=w1938) -> (.not. x?=w1937:bool)
                }
              }
            }
            n1268 = Not(x=w1891) -> (.not. x?=w1890:bool)
            n1269 = case shown="True" w1890 {
              tunnel: w1888 -> [_ w1954]
              tunnel: w1886 -> [_ w1953]
              tunnel: w1889 -> [_ w1952]
              tunnel: w1887 -> [_ w1951]
              frame False {
              }
              frame True {
                w1947 = FALSE ("Get Point")
                n1270 = local read "Scan lines (y)"() -> (w1956:u64)
                n1271 = local read "Actual MCL Inc (V)"() -> (w1948:dbl)
                n1272 = local read "Scan steps (MCL)"() -> (w1955:u64)
                n1273 = Divide "Y Pix/step"(x=w1951, y=w1956) -> (x/y=w1963:dbl)
                n1274 = Divide "Y V/pix"(x=w1948, y=w1963) -> (x/y=w1962:dbl)
                n1275 = Divide "Y half step offset"(x=w1948, y=2.0) -> (x/y=w1964:dbl)
                n1276 = Divide "X pix/step"(x=w1952, y=w1955) -> (x/y=w1961:dbl)
                n1277 = Negate(x=w1964) -> (-x=w1965:dbl)
                n1278 = local read "Initial Y"() -> (w1971:dbl)
                n1279 = Multiply(x=w1953, y=w1962) -> (x*y=w1972:dbl)
                n1280 = Divide "X half step offset"(x=w1948, y=2.0) -> (x/y=w1958:dbl)
                n1281 = Divide "X V/pix"(x=w1948, y=w1961) -> (x/y=w1960:dbl)
                n1282 = Multiply(x=w1948, y=w1955) -> (x*y=w1967:dbl)
                n1283 = Compound Arithmetic op=ADD(w1965, w1972, w1971) -> (w1949:dbl)
                "Pointer Y (V)" <- w1949
                n1284 = Multiply(x=w1960, y=w1954) -> (x*y=w1969:dbl)
                n1285 = Negate(x=w1958) -> (-x=w1957:dbl)
                n1286 = local read "Initial X"() -> (w1970:dbl)
                n1287 = Negate(x=w1969) -> (-x=w1968:dbl)
                n1288 = Compound Arithmetic op=ADD(w1957, w1967, w1970, w1968) -> (w1950:dbl)
                "Pointer X (V)" <- w1950
                n1289 = Or(x="Set X Only", y="Set Confocal Spot (X-Y)") -> (x .or. y?=w1943:bool)
                n1290 = Or(x="Set Confocal Spot (X-Y)", y="Set Y Only") -> (x .or. y?=w1942:bool)
                n1291 = case shown="True" w1943 {
                  tunnel: w1950 -> [_ w1973]
                  frame False {
                  }
                  frame True {
                    n1292 = property on="AO2" class="Slide (strict)"("Val(Sgnl)"=w1973) -> ()  [unwired: 2 in, 2 out]
                  }
                }
                n1293 = case shown="True" w1942 {
                  tunnel: w1949 -> [_ w1974]
                  frame False {
                  }
                  frame True {
                    n1294 = property on="AO1" class="Slide (strict)"("Val(Sgnl)"=w1974) -> ()  [unwired: 2 in, 2 out]
                  }
                }
                n1295 = local write "Set Confocal Spot (X-Y)"(w1947) -> ()
                n1296 = local write "Set X Only"(w1947) -> ()
                n1297 = local write "Set Y Only"(w1947) -> ()
              }
            }
          }
          frame 3 {
            n1298 = local read "BD 2 Frequency 1 (MHz)"() -> (w1975:dbl)
            n1299 = local read "BD 1 Frequency 1 (MHz)"() -> (w1976:dbl)
